vi "MQTT_Read_Published_Message.vi"(8 "error in (no error)":errorcluster, 11 "connection ID":refnum<k5>) -> (0 "error out":errorcluster, 1 "Message":string="MQIsdp", 2 "Topic Name":string="Topic", 3 "connection ID out":refnum<k5>, 4 "MessageType":T1, 5 "Message ID":u16=1 format="%x")   [LabVIEW 2025, in "MQTT_Functions.lvlib"]
doc: "This VI reads the last published message at the selected topic. It sends acknowledge information if required by the QoS level.\n\n© 2015 - daq.io, LLC - Peter Adelhardt"
uses:
  MQTT_Functions.lvlib
  Controls/MessageType.ctl
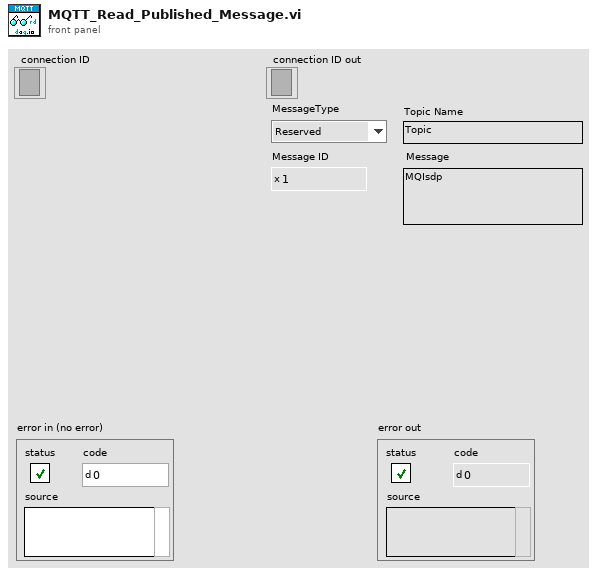
[diagram p1: front panel]
types:
  T1 = typedef "MQTT_Functions.lvlib/MessageType.ctl" = enum32{"Reserved", "CONNECT", "CONNACK", "PUBLISH", "PUBACK", "PUBREC", "PUBREL", "PUBCOMP", "SUBSCRIBE", "SUBACK", "UNSUBSCRIBE", "UNSUBACK", "PINGREQ", "PINGRESP", "DISCONNECT", "Reserved2"}
  T2 = typedef "MQTT_Functions.lvlib/QoS.ctl" = enum8{"At most once", "At least once", "Exactly once", "Reserved"}
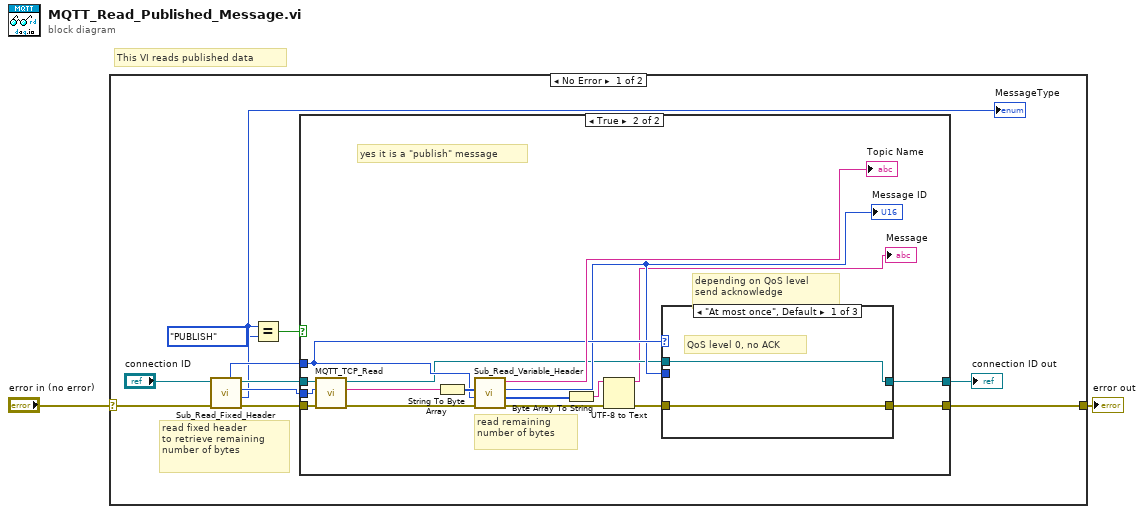
[diagram p0: block diagram]
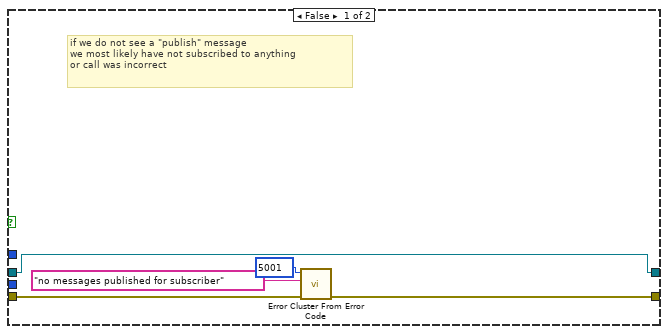
[diagram p2: hidden frame]
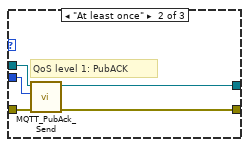
[diagram p3: hidden frame]
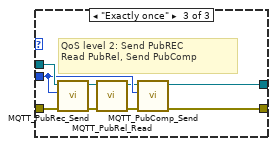
[diagram p4: hidden frame]
diagram:
  # "This VI reads published data"
  n1 = case shown="No Error" "error in (no error)" {
    selector: "error in (no error)" -> [w12 w52]
    tunnel: [w6 w52] -> w1
    frame No Error {
      # "read fixed header \nto retrieve remaining\nnumber of bytes"
      n2 = call "Sub_Read_Fixed_Header.vi"("error in (no error)"=w12, "connection ID"="connection ID") -> ("error out"=w9:errorcluster, "MessageType"=w5:T1, "Remaining Length"=w11:u32, "connection ID out"=w10:refnum<k5>, "QoS Level"=w8:T2)  [unwired: 3 in, 2 out]
      "MessageType" <- w5
      n3 = Equal?(x=w5, y=MessageType."PUBLISH") -> (x = y?=w3:bool)
      n4 = case shown="True" w3 {
        tunnel: w11 -> [_ w34]
        tunnel: w10 -> [w14 w33]
        tunnel: w9 -> [w18 w32]
        tunnel: w8 -> [_ w28]
        tunnel: [w14 w25] -> w7
        tunnel: [w15 w24] -> w6
        frame False {
          # "if we do not see a \"publish\" message\nwe most likely have not subscribed to anything\nor call was incorrect"
          n5 = call <vilib>:"Error Cluster From Error Code.vi"("error in (no error)"=w18, "error message (\"\")"="no messages published for subscriber" ("error message (\"\")"), "error code (0)"=5001) -> ("error out"=w15:errorcluster)  [unwired: 6 in]
        }
        frame True {
          # "yes it is a \"publish\" message"
          # "depending on QoS level\nsend acknowledge"
          # "read remaining\nnumber of bytes"
          n6 = call "MQTT_TCP_Read.vi"("error in (no error)"=w32, "bytes to read"=w34, "connection ID"=w33) -> ("error out"=w29:errorcluster, "data out"=w31:string, "connection ID out"=w26:refnum<k5>)  [unwired: 6 in]
          n7 = String To Byte Array(string=w31) -> (unsigned byte array=w30:u8[])
          n8 = call "Sub_Read_Variable_Header.vi"("error in (no error)"=w29, "QoS"=w28, "Variable Header"=w30) -> ("error out"=w19:errorcluster, "remaining bytes"=w23:u8[], "Message ID"=w27:u16, "Topic Name"=→"Topic Name":string)  [unwired: 5 in]
          "Message ID" <- w27
          n9 = Byte Array To String(unsigned byte array=w23) -> (string=w22:string)
          n10 = UTF-8 to Text(8:w19, 11:w22) -> (0:w20:errorcluster, 3:→"Message":string)  [unwired: 1 in]
          n11 = case shown="\"At most once\", Default" w28 {
            tunnel: w27 -> [_ w42 w47]
            tunnel: w20 -> [w36 w41 w51]
            tunnel: w26 -> [w37 w40 w50]
            tunnel: [w37 w39 w49] -> w25
            tunnel: [w36 w38 w48] -> w24
            frame "At most once", Default {
              # "QoS level 0, no ACK"
            }
            frame "At least once" {
              # "QoS level 1: PubACK"
              n12 = call "MQTT_PubAck_Send.vi"("error in (no error)"=w41, "Message ID"=w42, "connection ID"=w40) -> ("error out"=w38:errorcluster, "connection ID out"=w39:refnum<k5>)  [unwired: 6 in, 1 out]
            }
            frame "Exactly once" {
              # "QoS level 2: Send PubREC\nRead PubRel, Send PubComp"
              n13 = call "MQTT_PubRec_Send.vi"("error in (no error)"=w51, "Message ID"=w47, "connection ID"=w50) -> ("error out"=w44:errorcluster, "connection ID out"=w43:refnum<k5>)  [unwired: 6 in, 1 out]
              n14 = call "MQTT_PubRel_Read.vi"("error in (no error)"=w44, "connection ID"=w43) -> ("error out"=w45:errorcluster, "connection ID out"=w46:refnum<k5>)  [unwired: 7 in, 1 out]
              n15 = call "MQTT_PubComp_Send.vi"("error in (no error)"=w45, "Message ID"=w47, "connection ID"=w46) -> ("error out"=w48:errorcluster, "connection ID out"=w49:refnum<k5>)  [unwired: 6 in, 1 out]
            }
          }
        }
      }
      "connection ID out" <- w7
    }
    frame Error {
    }
  }
  "error out" <- w1
